vi "Update Graphs.vi"(8 "error in (no error)":errorcluster, 11 "Sensor & Control in":refnum<class "Control.lvclass">) -> (0 "error out":errorcluster, 3 "Sensor & Control out":refnum<class "Control.lvclass">)   [LabVIEW 2013, in "Control.lvib.lvlib" / "Control.lvclass"]
uses:
  Control.lvclass
  Control.lvclass/Control.ctl
  Read Graph History.vi
  Read Graph.vi
  Read Setpoint.vi
  PluginInterface/PluginInterface.lvlibp/PluginInterfaceClass/Read TDMS.vi
  PluginInterface/PluginInterface.lvlibp/PluginInterfaceClass/Read Name.vi
  PluginInterface/PluginInterface.lvlibp/PluginInterfaceClass/Read DVR.vi
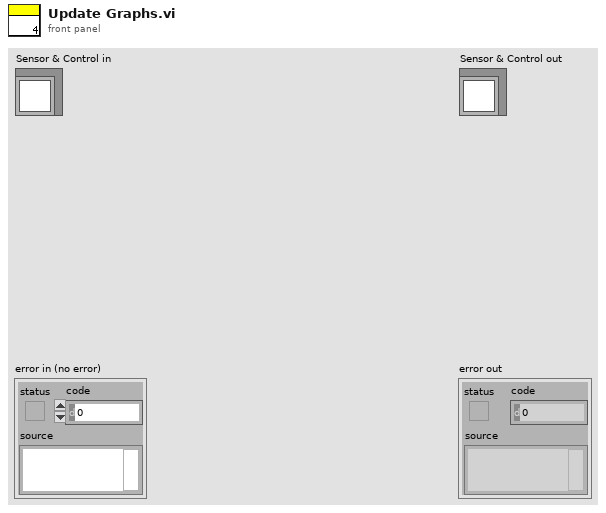
[diagram p1: front panel]
types:
  T1 = cluster{"output array":dbl[], "output array":dbl[]}
  T2 = cluster{"output array":dbl[], "output array":dbl[]}[]
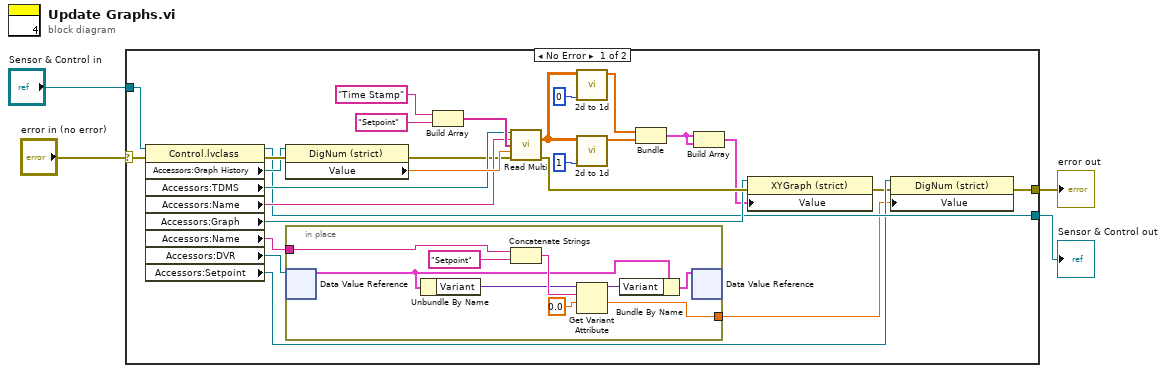
[diagram p0: block diagram]
diagram:
  n1 = case shown="No Error" "error in (no error)" {
    selector: "error in (no error)" -> [w28 w42]
    tunnel: [w6 w42] -> w1
    tunnel: [w13 w41] -> w2
    tunnel: "Sensor & Control in" -> [w31 w41]
    frame No Error {
      n2 = property class="Control.lvclass"(reference=w31, error in=w28) -> (reference out=w13:refnum<class "Control.lvclass">, error out=w27:errorcluster, "Accessors:Graph History"=w23:refnum<vi>, "Accessors:TDMS"=w24:refnum<k34>, "Accessors:Name"=w15:string, "Accessors:Graph"=w21:refnum<vi>, "Accessors:Name"=w10:string, "Accessors:DVR"=w9:refnum<data-value>, "Accessors:Setpoint"=w8:refnum<vi>)
      n3 = property class="DigNum (strict)"(reference=w23, error in=w27) -> (error out=w14:errorcluster, "Value"=w25:dbl)  [unwired: 1 out]
      n4 = in-place {
        in-place-border: w10 -> [w40]
        in-place-border: [w39] -> w5
        n5 = in-place-dvr #1(w9) -> (w35:cluster{"Array":string[], "Variant":variant})  [unwired: 1 out]
        n6 = Unbundle By Name(w35) -> ("Variant"=w34:variant)
        n7 = Concatenate Strings(w40, "Setpoint" ("string")) -> (w36:string)
        n8 = Get Variant Attribute(Variant=w34, name=w36, default value (empty Variant)=0.0 ("Value")) -> (duplicate Variant=w33:variant, value=w39:dbl)  [unwired: 1 in, 2 out]
        n9 = Bundle By Name(cluster=w35, "Variant"=w33) -> (w32:cluster{"Array":string[], "Variant":variant})
        n10 = in-place-dvr #1(w32) -> ()  [unwired: 2 out]
      }
      n11 = Build Array("Time Stamp" ("Channel"), "Setpoint" ("string")) -> (w26:string[])
      n12 = call "Read Multi.vi"("tdms file in"=w24, "group"=w15, "Channel"=w26, "Numeric"=w25, "error in (no error)"=w14) -> ("Array"=w17:dbl[][], "error out"=w22:errorcluster)  [unwired: 7 in, 2 out]
      n13 = call "2d to 1d.vi"("index"=0, "array"=w17) -> ("output array"=w18:dbl[])  [unwired: 9 in]
      n14 = call "2d to 1d.vi"("index"=1, "array"=w17) -> ("output array"=w16:dbl[])  [unwired: 9 in]
      n15 = Bundle("output array"=w18, "output array"=w16) -> (w12:T1)  [unwired: 1 in]
      n16 = Build Array(w12, w12) -> (w11:T2)
      n17 = property class="XYGraph (strict)"(reference=w21, error in=w22, "Value"=w11) -> (error out=w7:errorcluster)  [unwired: 1 out]
      n18 = property class="DigNum (strict)"(reference=w8, error in=w7, "Value"=w5) -> (error out=w6:errorcluster)  [unwired: 1 out]
    }
    frame Error {
    }
  }
  "error out" <- w1
  "Sensor & Control out" <- w2
